vi "free index.vi"(0 "index_id":u64, 3 "Overwrite Lib Path":path, 9 "flann_params":T1 {"algorithm" items=["FLANN_INDEX_LINEAR"=0, "FLANN_INDEX_KDTREE"=1, "FLANN_INDEX_KMEANS"=2, "FLANN_INDEX_COMPOSITE"=3, "FLANN_INDEX_KDTREE_SINGLE"=4, "FLANN_INDEX_HIERARCHICAL"=5, "FLANN_INDEX_LSH"=6, "FLANN_INDEX_SAVED"=254, "FLANN_INDEX_AUTOTUNED"=255]; "centers_init" items=["FLANN_CENTERS_RANDOM", "FLANN_CENTERS_GONZALES", "FLANN_CENTERS_KMEANSPP", "FLANN_CENTERS_GROUPWISE"]; "log_level" items=["FLANN_LOG_NONE", "FLANN_LOG_FATAL", "FLANN_LOG_ERROR", "FLANN_LOG_WARN", "FLANN_LOG_INFO", "FLANN_LOG_DEBUG"]}, 11 "error in (no error)":errorcluster) -> (10 "function return":i32, 15 "error out":errorcluster)   [LabVIEW 2020, in "KD Tree.lvlib"]
doc: "FLANN_EXPORT int flann_free_index(flann_index_t index_id,\n struct FLANNParameters* flann_params);"
uses:
  KD Tree.lvlib
  Flann Params.ctl
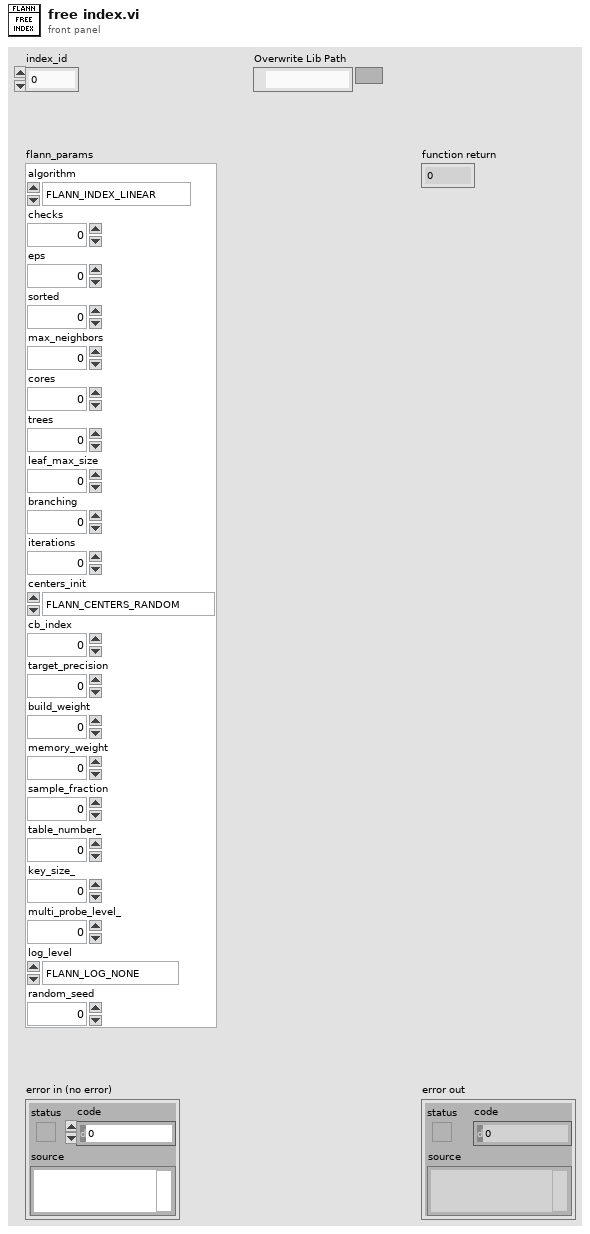
[diagram p1: front panel]
types:
  T1 = typedef "KD Tree.lvlib/Flann Params.ctl" = cluster{"algorithm":u32, "checks":i32, "eps":sgl, "sorted":i32, "max_neighbors":i32, "cores":i32, "trees":i32, "leaf_max_size":i32, "branching":i32, "iterations":i32, "centers_init":u32, "cb_index":sgl, "target_precision":sgl, "build_weight":sgl, "memory_weight":sgl, "sample_fraction":sgl, "table_number_":u32, "key_size_":u32, "multi_probe_level_":u32, "log_level":u32, "random_seed":i32}
  T2 = typedef "Semaphore RefNum" = refnum<k1>
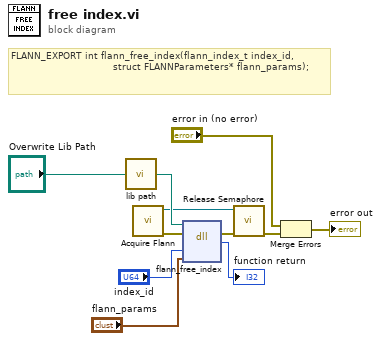
[diagram p0: block diagram]
diagram:
  # "FLANN_EXPORT int flann_free_index(flann_index_t index_id,\n                                  struct FLANNParameters* flann_params);"
  n1 = call "lib path.vi"("Overwrite Lib Path"="Overwrite Lib Path") -> ("lib path"=w7:path)
  n2 = call "Acquire Flann.vi"() -> ("error out"=w1:errorcluster, "semaphore"=w2:T2)  [unwired: 10 in]
  n3 = dll-call lib="E:/Labview/LV 2020/Libs/flann/flann.dll" fn="flann_free_index"(path in=w7, error in=w1, "index_id"="index_id", "flann_params"="flann_params") -> (error out=w8:errorcluster, "return type"=→"function return":i32)  [unwired: 3 in, 1 out]
  n4 = call <vilib>:"Release Semaphore.vi"("error in (no error)"=w8, "semaphore"=w2) -> ("error out"=w3:errorcluster)  [unwired: 4 in, 1 out]
  n5 = Merge Errors("error in (no error)", w3) -> (→"error out":errorcluster)
